vi "RampPower.vi"(6 "Auto Range Terminal":i32(ring) items=["Low", "High"], 8 "Error In":errorcluster, 9 "Cluster":T2={"milliseconds to wait"=30, "deltaV"=0.2, "Vhigh"=1.6, "Vlow"=0.0}, 10 "Power Channel":tag="VB8012-3060439/ps/+6V", 11 "Instrument Handles":T1) -> (0 "Error Out":errorcluster={"status"=TRUE, "code"=-375945, "source"="VirtualBench.lvlib:PS Read Output.vi:5070001<append>\n"}, 2 "Voltage & Current":cluster{dbl[], dbl[]}, 3 "PWS Out":refnum<k21>="_ps3")   [LabVIEW 2015]
uses:
  <vilib>/Analysis/1siggen.llb/Ramp Pattern by Delta.vi
  <vilib>/VirtualBench/_DMM Configure Measurement4.vi
  <vilib>/VirtualBench/_PS Configure Voltage Output2.vi
  <vilib>/Analysis/NI_AALBase.lvlib
  <vilib>/VirtualBench/VirtualBench.lvlib
panel:
  # "t"
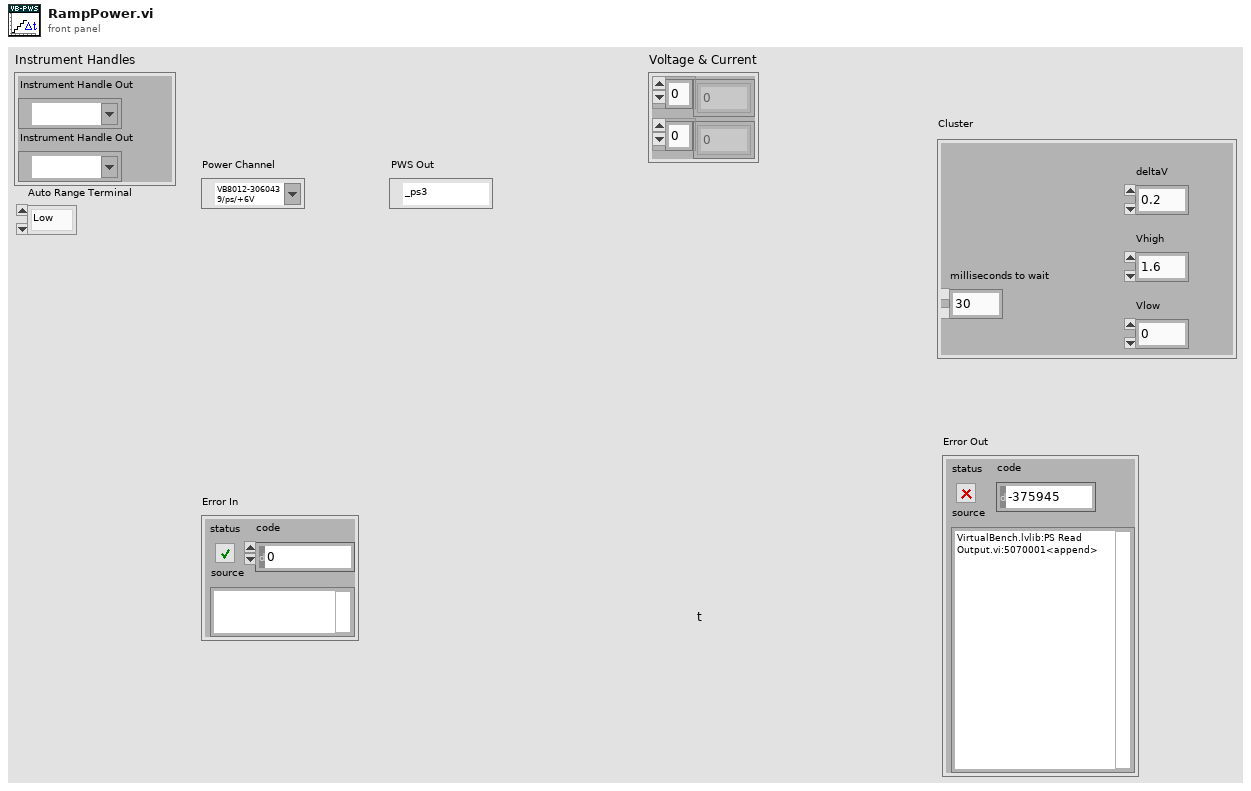
[diagram p1: front panel]
types:
  T1 = cluster{"Instrument Handle Out":refnum<k21>, "Instrument Handle Out":refnum<k21>}
  T2 = cluster{"milliseconds to wait":u32, "deltaV":dbl, "Vhigh":dbl, "Vlow":dbl}
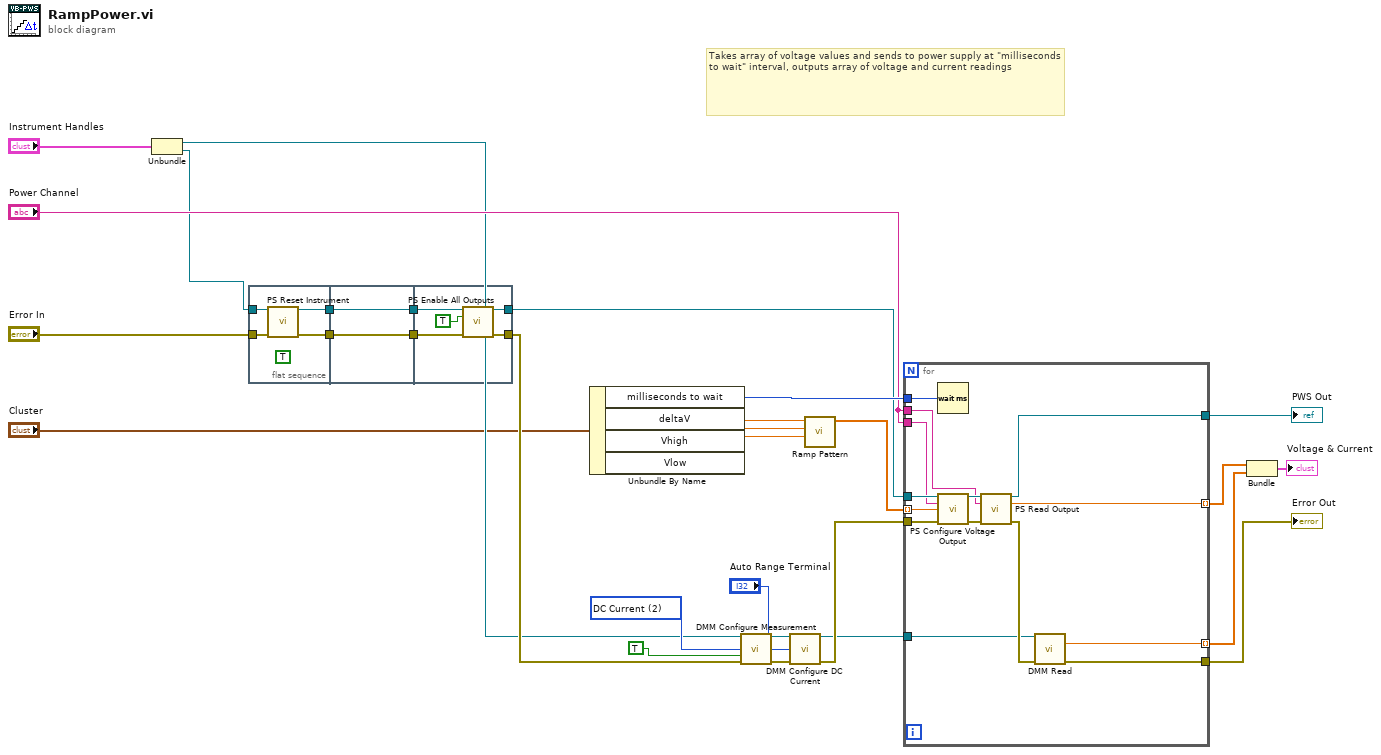
[diagram p0: block diagram]
diagram:
  w13 = 2 items=["DC Volts", "AC Volts", "DC Current", "AC Current", "Resistance", "Diode"] ("Function")
  # "Takes array of voltage values and sends to power supply at \"milliseconds to wait\" interval, outputs array of voltage and current readings"
  n1 = Unbundle("Instrument Handles") -> ("Instrument Handle Out"=w7:refnum<k21>, "Instrument Handle Out"=w8:refnum<k21>)
  n2 = flat-sequence {
    tunnel: [w33] -> w21
    tunnel: [w32] -> w19
    tunnel: w8 -> [w31]
    tunnel: "Error In" -> [w30]
    tunnel: [w35] -> w22
    tunnel: w21 -> [w35]
    tunnel: [w34] -> w20
    tunnel: w19 -> [w34]
    tunnel: w22 -> [w40]
    tunnel: w20 -> [w39]
    tunnel: [w38] -> w18
    tunnel: [w36] -> w11
    frame #0 {
      (unwired) TRUE ("Enable Outputs")
      n3 = call <vilib>:"PS Reset Instrument.vi"("Instrument Handle In"=w31, "Error In"=w30) -> ("Instrument Handle Out"=w33:refnum<k21>, "Error Out"=w32:errorcluster)  [unwired: 12 in]
    }
    frame #1 {
    }
    frame #2 {
      n4 = call <vilib>:"PS Enable All Outputs.vi"("Instrument Handle In"=w40, "Enable Outputs"=TRUE, "Error In"=w39) -> ("Instrument Handle Out"=w38:refnum<k21>, "Error Out"=w36:errorcluster)  [unwired: 11 in]
    }
  }
  n5 = Unbundle By Name("Cluster") -> ("milliseconds to wait"=w25:u32, "deltaV"=w28:dbl, "Vhigh"=w27:dbl, "Vlow"=w26:dbl)
  n6 = call-poly <vilib>:"DMM Configure Measurement.vi"("Instrument Handle In"=w7, "Function"=w13, "Auto Range"=TRUE, "Error In"=w11) -> ("Instrument Handle Out"=w5:refnum<k21>, "Error Out"=w4:errorcluster)  [unwired: 10 in]
  n7 = call <vilib>:"DMM Configure DC Current.vi"("Instrument Handle In"=w5, "Auto Range Terminal"="Auto Range Terminal", "Error In"=w4) -> ("Instrument Handle Out"=w2:refnum<k21>, "Error Out"=w3:errorcluster)  [unwired: 11 in]
  n8 = call-poly <vilib>:"Ramp Pattern.vi"("start"=w26, "end"=w27, "delta"=w28) -> ("Ramp Pattern"=w29:dbl[])  [unwired: 6 in, 2 out]
  n9 = for {
    tunnel: w29 -> [w52] mode=indexing
    tunnel: [w51] -> w24
    tunnel: w25 -> [w50]
    tunnel: w18 -> [w49]
    tunnel: "Power Channel" -> [w48]
    tunnel: w3 -> [w47]
    tunnel: "Power Channel" -> [w46]
    tunnel: [w43] -> w16 mode=indexing
    tunnel: [w45] -> w15 mode=indexing
    tunnel: w2 -> [w42]
    tunnel: [w41] -> w10
    n10 = Wait (ms)(milliseconds to wait=w50) -> ()  [unwired: 1 out]
    n11 = call-poly <vilib>:"PS Configure Voltage Output.vi"("Instrument Handle In"=w49, "Channel"=w48, "Voltage Level"=w52, "Error In"=w47) -> ("Instrument Handle Out"=w54:refnum<k21>, "Error Out"=w53:errorcluster)  [unwired: 10 in]
    n12 = call <vilib>:"PS Read Output.vi"("Instrument Handle In"=w54, "Channel"=w46, "Error In"=w53) -> ("Instrument Handle Out"=w51:refnum<k21>, "Actual Voltage Level"=w43:dbl, "Error Out"=w44:errorcluster)  [unwired: 8 in, 2 out]
    n13 = call <vilib>:"DMM Read.vi"("Instrument Handle In"=w42, "Error In"=w44) -> ("Measurement"=w45:dbl, "Error Out"=w41:errorcluster)  [unwired: 11 in, 1 out]
  }
  "PWS Out" <- w24
  "Error Out" <- w10
  n14 = Bundle(w16, w15) -> (→"Voltage & Current":cluster{dbl[], dbl[]})  [unwired: 1 in]
